vi "ForveWhileKullanarakRasgeleSayılarıDiziye kaydetme.vi"() -> ()   [LabVIEW 2014]
panel:
  out "Array 2":dbl[](array[numeric])
  out "Array":dbl[](array[numeric])
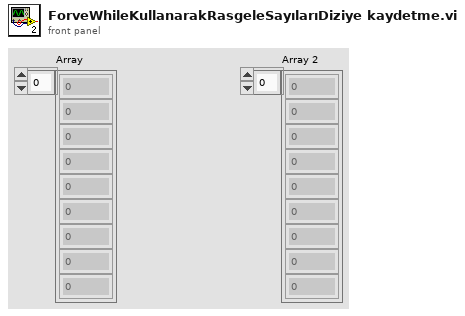
[diagram p1: front panel]
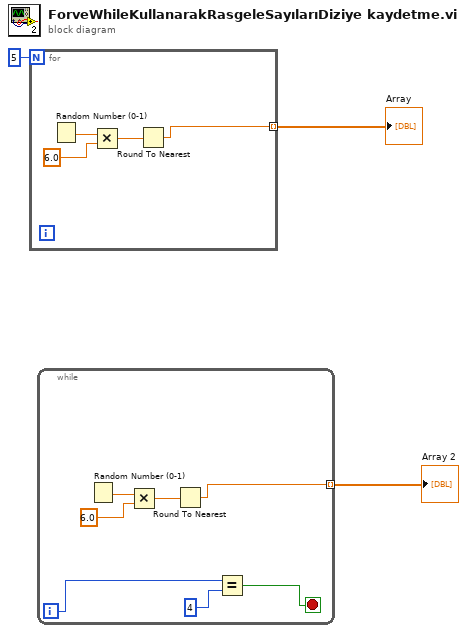
[diagram p0: block diagram]
diagram:
  n1 = for {
    N: 5 -> [_]
    tunnel: [w4] -> w2 mode=indexing
    n2 = Random Number (0-1)() -> (number: 0 to 1=w7:dbl)
    n3 = Multiply(x=w7, y=6.0) -> (x*y=w5:dbl)
    n4 = Round To Nearest(number=w5) -> (nearest integer value=w4:dbl)
  }
  "Array" <- w2
  n5 = while {
    tunnel: [w8] -> w1 mode=indexing
    i -> [w11]
    stop <- w9 stop-if-true
    n6 = Random Number (0-1)() -> (number: 0 to 1=w12:dbl)
    n7 = Multiply(x=w12, y=6.0) -> (x*y=w14:dbl)
    n8 = Round To Nearest(number=w14) -> (nearest integer value=w8:dbl)
    n9 = Equal?(x=w11, y=4) -> (x = y?=w9:bool)
  }
  "Array 2" <- w1
